vi "Add Series.vi"(8 "error in (no error)":errorcluster, 10 ".net MSChart Series":refnum<k24>, 11 ".NET MSChart":refnum<k24>) -> (0 "error out":errorcluster, 3 ".NET MSChart (dup)":refnum<k24>)   [LabVIEW 2014, in "XMSChart.xctl"]
uses:
  XMSChart.xctl
  System.Windows.Forms.DataVisualization
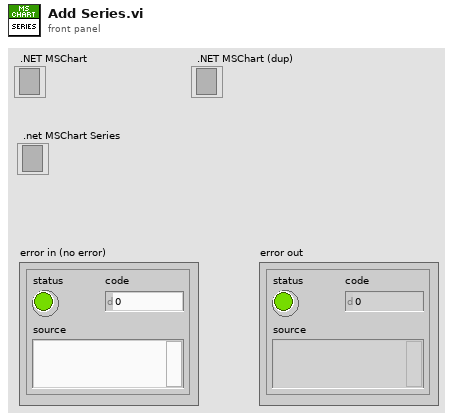
[diagram p1: front panel]
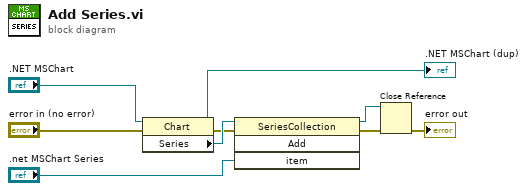
[diagram p0: block diagram]
diagram:
  n1 = property class="Chart"(reference=".NET MSChart", error in="error in (no error)") -> (reference out=→".NET MSChart (dup)":refnum<k24>, error out=w6:errorcluster, "Series"=w7:refnum<k24>)
  n2 = invoke class="SeriesCollection" method="Add"(reference=w7, error in=w6, "item"=".net MSChart Series") -> (reference out=w2:refnum<k24>, error out=w5:errorcluster)  [unwired: 1 in, 2 out]
  n3 = Close Reference(reference=w2, error in (no error)=w5) -> (error out=→"error out":errorcluster)
